vi "LIN UDS Get Msg From UDS Buffer.vi"(7 "BufferSize":i32, 8 "error in (no error)":errorcluster, 9 "pCanGetMsg":T1, 10 "LINIndex":u8, 11 "DevHandle":i32) -> (0 "error out":errorcluster, 1 "pCanGetMsg out":T1, 3 "function return":i32)   [LabVIEW 2010, in "lin_uds.lvlib"]
doc: "int WINAPI LIN_UDS_GetMsgFromUDSBuffer(int DevHandle,unsigned char LINIndex,LIN_EX_MSG *pCanGetMsg,int BufferSize);"
uses:
  lin_uds.lvlib
  USB2XXX/trunk/USB2XXX/USB2XXX/vs2010/Release/USB2XXX.dll
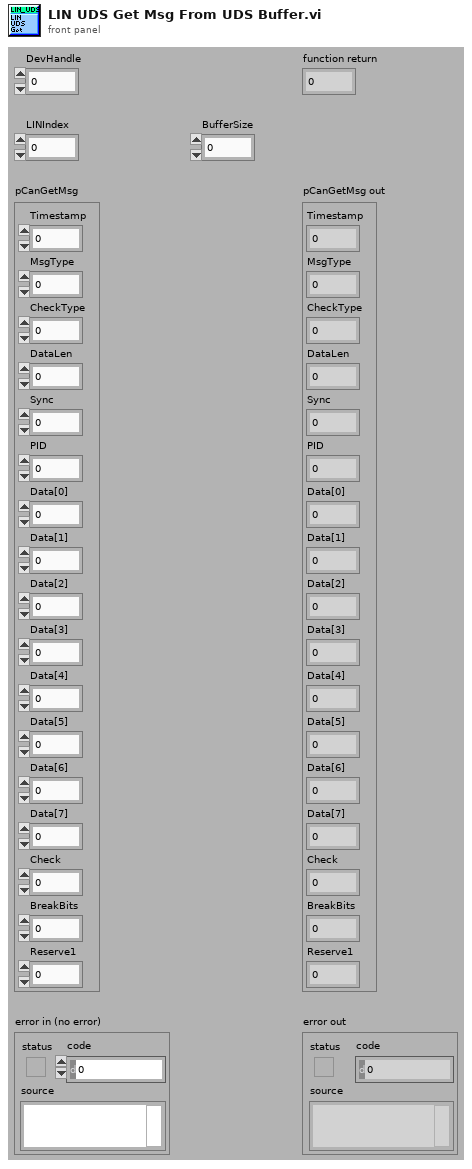
[diagram p1: front panel]
types:
  T1 = cluster{"Timestamp":u32, "MsgType":u8, "CheckType":u8, "DataLen":u8, "Sync":u8, "PID":u8, "Data[0]":u8, "Data[1]":u8, "Data[2]":u8, "Data[3]":u8, "Data[4]":u8, "Data[5]":u8, "Data[6]":u8, "Data[7]":u8, "Check":u8, "BreakBits":u8, "Reserve1":u8}
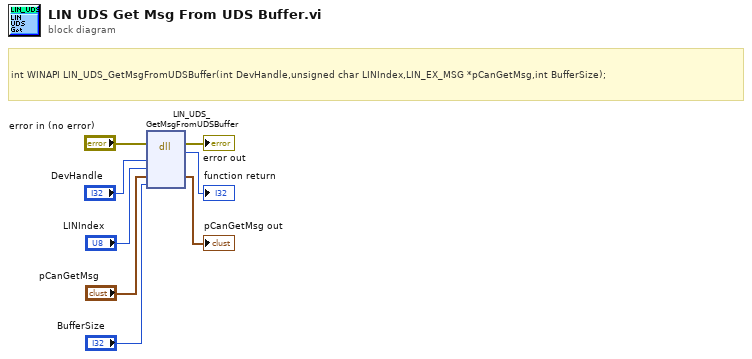
[diagram p0: block diagram]
diagram:
  # "int WINAPI LIN_UDS_GetMsgFromUDSBuffer(int DevHandle,unsigned char LINIndex,LIN_EX_MSG *pCanGetMsg,int BufferSize);"
  n1 = dll-call lib="E:/OtherWork/STM32/USB2XXX/trunk/USB2XXX/USB2XXX/vs2010/Release/USB2XXX.*" fn="LIN_UDS_GetMsgFromUDSBuffer"(error in="error in (no error)", "DevHandle"="DevHandle", "LINIndex"="LINIndex", "pCanGetMsg"="pCanGetMsg", "BufferSize"="BufferSize") -> (error out=→"error out":errorcluster, →"function return":i32, "pCanGetMsg"=→"pCanGetMsg out":T1)  [unwired: 5 in, 1 out]
